vi "testScriptingImportSendUDP.vi"(8 "error in (no error)":errorcluster, 11 "TestCase in":refnum<class "Scripting.lvclass">) -> (0 "error out":errorcluster, 3 "TestCase out":refnum<class "Scripting.lvclass">)   [LabVIEW 2019, in "Scripting.lvclass"]
uses:
  Scripting.lvclass
  <vilib>/addons/_JKI Toolkits/VI Tester/TestCase.llb/TestCase.lvclass
  <vilib>/NI VeriStand/Execution/Workspace/NI_VS Workspace ExecutionAPI.lvlib
  b55b5565-dc34-4e51-bcfa-5a6cba25043e.vi
  <vilib>/NI VeriStand/Execution/Workspace/NI VeriStand - Set Multiple Channel Values.vi
  Scripting Examples/Data Sharing Framework Scripting Examples.lvlib
  C:/Program Files (x86)/National Instruments/LabVIEW 2017/vi.lib/addons/_JKI Toolkits/VI Tester/TestCase.llb/TestCase.lvclass
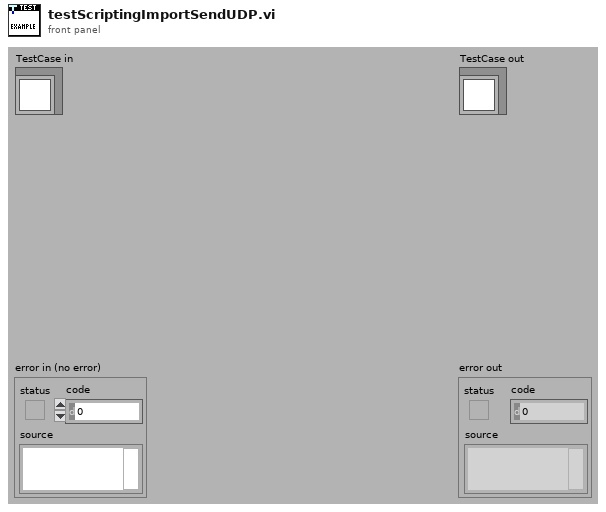
[diagram p1: front panel]
types:
  T1 = typedef "NI_VS Workspace ExecutionAPI.lvlib/WorkspaceAPI.ctl" = refnum<k24>
  T2 = typedef "NI_VS Workspace ExecutionAPI.lvlib/NodeInfo.ctl" = cluster{"Name":string, "FullPath":string, "Type":string, "IsChannel":bool, "Channel":cluster{"Unit":string, "Readable":bool, "Writable":bool, "Faultable":bool, "Scalable":bool, "RowDim":u32, "ColumnDim":u32, "Value Table Names":string[], "Value Table Values":dbl[]}, "IsWaveform":bool, "Waveform":cluster{"DataType":T3}}
  T3 = typedef "NI_VS Workspace ExecutionAPI.lvlib/Waveform Data Type.ctl" = enum16{"Double", "ComplexDouble"}
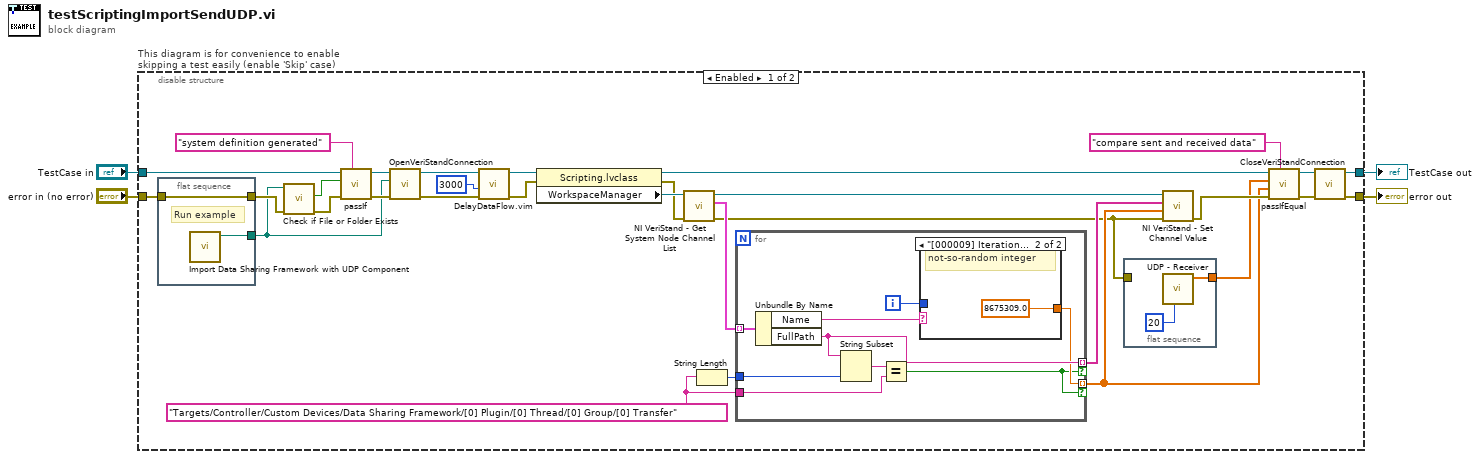
[diagram p0: block diagram]
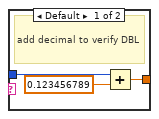
[diagram p2: hidden frame]
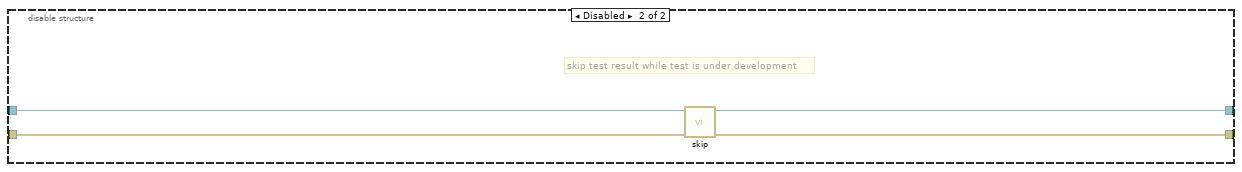
[diagram p3: hidden frame]
diagram:
  n1 = disable-structure "This diagram is for convenience to enable skipping a test easily (enable 'Skip' case)" shown="Enabled" {
    disable-tunnel: "TestCase in" -> [w19 w55]
    disable-tunnel: [w28 w53] -> w1
    disable-tunnel: [w26 w54] -> w2
    disable-tunnel: "error in (no error)" -> [w25 w52]
    frame Enabled {
      w15 = "Targets/Controller/Custom Devices/Data Sharing Framework/[0] Plugin/[0] Thread/[0] Group/[0] Transfer" ("FullPath")
      n2 = flat-sequence {
        tunnel: w25 -> [w51]
        tunnel: [w51] -> w17
        tunnel: [w50] -> w7
        frame #0 {
          # "Run example"
          n3 = call "Import Data Sharing Framework with UDP Component.vi"() -> ("Output System Definition File"=w50:path)  [unwired: 11 in]
        }
      }
      n4 = call <vilib>:"Check if File or Folder Exists.vi"("error in (no error)"=w17, "path"=w7) -> ("error out"=w8:errorcluster, "file or folder exists?"=w21:bool)  [unwired: 7 in, 1 out]
      n5 = call-dynamic "passIf.vi"("custom report message (\"\")"="system definition generated" ("custom report message (\"\")"), "error in (no error)"=w8, "pass"=w21, "TestCase in"=w19) -> ("error out"=w20:errorcluster, "TestCase out"=w18:refnum<class "Scripting.lvclass">)  [unwired: 6 in]
      n6 = call-dynamic "OpenVeriStandConnection.vi"("error in (no error)"=w20, "System Definition File"=w7, "VeriStand Test Case in"=w18) -> ("error out"=w31:errorcluster, "VeriStand Test Case out"=w34:refnum<class "Scripting.lvclass">)  [unwired: 6 in, 1 out]
      n7 = call "DelayDataFlow.vim"("value in"=w31, "milliseconds to wait"=u32 3000) -> ("value out"=w30:errorcluster)  [unwired: 2 in, 1 out]
      n8 = property class="Scripting.lvclass"(reference=w34, error in=w30) -> (reference out=w33:refnum<class "Scripting.lvclass">, error out=w22:errorcluster, "WorkspaceManager"=w24:T1)
      n9 = call <vilib>:"NI VeriStand - Get System Node Channel List.vi"("error in (no error)"=w22, "WorkspaceManager in"=w24) -> ("error out"=w5:errorcluster, "Channels"=w14:T2[], "WorkspaceManager out"=w23:T1)  [unwired: 7 in]
      n10 = String Length(string=w15) -> (length=w16:i32)
      n11 = for {
        tunnel: w14 -> [w45] mode=indexing
        tunnel: w16 -> [w44]
        tunnel: w15 -> [w43]
        tunnel: [w40] -> w13 mode=indexing if=w37
        tunnel: [w38] -> w10 mode=indexing if=w37
        i -> [w39]
        n12 = Unbundle By Name(w45) -> ("Name"=w41:string, "FullPath"=w40:string)
        n13 = String Subset(string=w40, length (rest)=w44) -> (substring=w42:string)  [unwired: 1 in]
        n14 = Equal?(x=w42, y=w43) -> (x = y?=w37:bool)
        n15 = case shown="\"[000009] Iterations\"" w41 {
          tunnel: w39 -> [w48 _]
          tunnel: [w46 8675309.0 ("Jenny")] -> w38
          frame Default {
            # "add decimal to verify DBL"
            n16 = Add(x=w48, y=0.123456789) -> (x+y=w46:dbl)
          }
          frame "[000009] Iterations" {
            # "not-so-random integer"
          }
        }
      }
      n17 = flat-sequence {
        tunnel: [w36] -> w6
        tunnel: w5 -> [_]
        frame #0 {
          n18 = call "UDP - Receiver.vi"("Maximum Iterations (-1=Inf)"=20 ("iterations (-1=Inf)")) -> ("Numerics (DBL)"=w36:dbl[])  [unwired: 10 in]
        }
      }
      n19 = call-poly <vilib>:"NI VeriStand - Set Channel Value.vi"("error in (no error)"=w5, "Values"=w10, "Channels"=w13, "WorkspaceManager in"=w23) -> ("error out"=w12:errorcluster)  [unwired: 6 in, 1 out]
      n20 = call-dynamic "passIfEqual.vi"("custom report message (\"\")"="compare sent and received data" ("custom report message (\"\")"), "error in (no error)"=w12, "y"=w10, "x"=w6, "TestCase in"=w33) -> ("error out"=w27:errorcluster, "TestCase out"=w29:refnum<class "Scripting.lvclass">)  [unwired: 5 in]
      n21 = call-dynamic "CloseVeriStandConnection.vi"("error in (no error)"=w27, "VeriStand Test Case in"=w29) -> ("error out"=w26:errorcluster, "VeriStand Test Case out"=w28:refnum<class "Scripting.lvclass">)  [unwired: 8 in]
    }
    frame Disabled {
      # "skip test result while test is under development"
      n22 = call <vilib>:"skip.vi"("error in (no error)"=w52, "TestCase in"=w55) -> ("error out"=w54:errorcluster, "TestCase out"=w53:refnum<class "Scripting.lvclass">)  [unwired: 8 in]
    }
  }
  "error out" <- w2
  "TestCase out" <- w1
